vi "write sequential I64s.vi"(9 "values":i64[](array[numeric]), 10 "index":i32, 11 "data table in":T1) -> (3 "data table out":T1)   [LabVIEW 2013, in "data bus values.lvlib"]
doc: "Writes a sequential set of data to the table."
uses:
  data bus values.lvlib
  data table.ctl
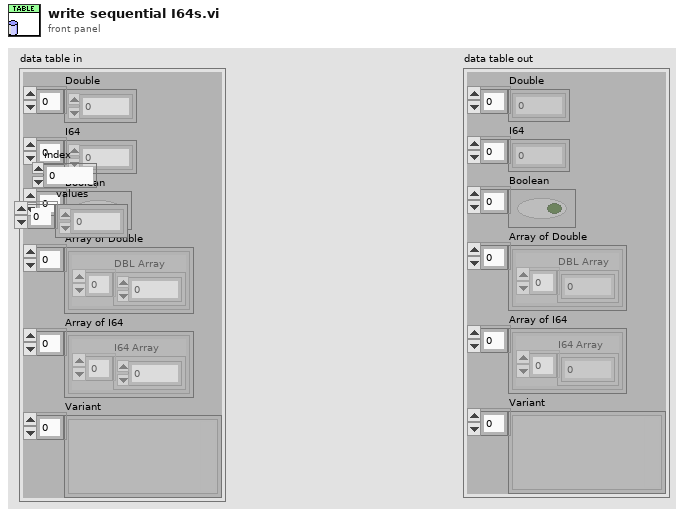
[diagram p1: front panel]
types:
  T1 = typedef "data bus values.lvlib/data table.ctl" = cluster{"Double":dbl[], "I64":i64[], "Boolean":bool[], "Array of Double":cluster{"DBL Array":dbl[]}[], "Array of I64":cluster{"I64 Array":i64[]}[], "Variant":variant[]}
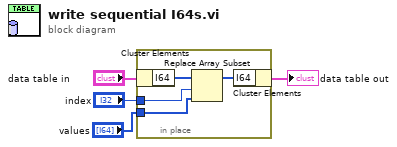
[diagram p0: block diagram]
diagram:
  n1 = in-place {
    in-place-border: "values" -> [w6]
    in-place-border: "index" -> [w5]
    n2 = in-place-cluster #1("data table in") -> ("I64"=w8:i64[])
    n3 = Replace Array Subset(array=w8, new element=w6, index=w5) -> (w7:i64[])
    n4 = in-place-cluster #1("I64"=w7) -> (→"data table out":T1)
  }
